vi "GetHelp.vi"(11 "PrintToSingleFileHtml in":refnum<class "PrintToSingleFileHtml.lvclass">) -> (2 "Help":string, 3 "PrintToSingleFileHtml out":refnum<class "PrintToSingleFileHtml.lvclass">)   [LabVIEW 2026, in "PrintToSingleFileHtml.lvclass"]
uses:
  PrintToSingleFileHtml.lvclass
  PrintToSingleFileHtml.lvclass/PrintToSingleFileHtml.ctl
panel:
  in  "help text":string="This operation takes a VI by name or path and prints its contents to an HTML file at the provided path. -o can be specified to overwrite if a report already exists at the report path. -c can be specified to create folders if the report path is under a non-existent path.\n\nExample: LabVIEWCLI -OperationName PrintToSingleFileHtml -VI VINameOrPath.vi -OutputPath ReportPath.html -o\n"
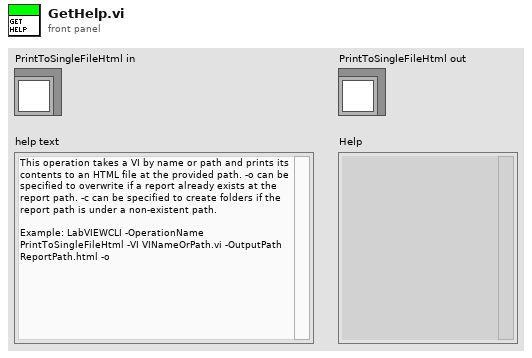
[diagram p1: front panel]
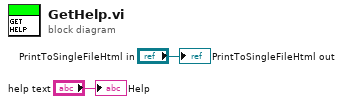
[diagram p0: block diagram]
diagram:
  "PrintToSingleFileHtml out" <- "PrintToSingleFileHtml in"
  "Help" <- "help text"
